vi "GetSignal.vi"(8 "error in (no error)":errorcluster, 11 "PmuTestFunctions in":refnum<class "PmuTestFunctions.lvclass">) -> (0 "error out":errorcluster, 2 "Signal":variant, 3 "PmuTestFunctions out":refnum<class "PmuTestFunctions.lvclass">)   [LabVIEW 2018, in "Functions.lvlib" / "PmuTestFunctions.lvclass"]
doc: "Gets the waveform, applies the gain and outputs a 2D array of the signal"
uses:
  PmuTestFunctions.lvclass
  X:/Projects/PMUCal/Modules/FGen/MemberClasses/FunctionBaseClass/FunctionBase.lvclass
  X:/Projects/PMUCal/Modules/FGen/MemberClasses/ArbitraryFunction/ArbitraryFunction.lvclass
  FunctionBaseClass/FunctionBase.lvclass/FunctionBase.ctl
  ArbitraryFunction/ArbitraryFunction.lvclass/ArbitraryFunction.ctl
  FunctionBaseClass/Accessors/Read Waveforms.vi
  ArbitraryFunction/Accessors/Read Arbs.vi
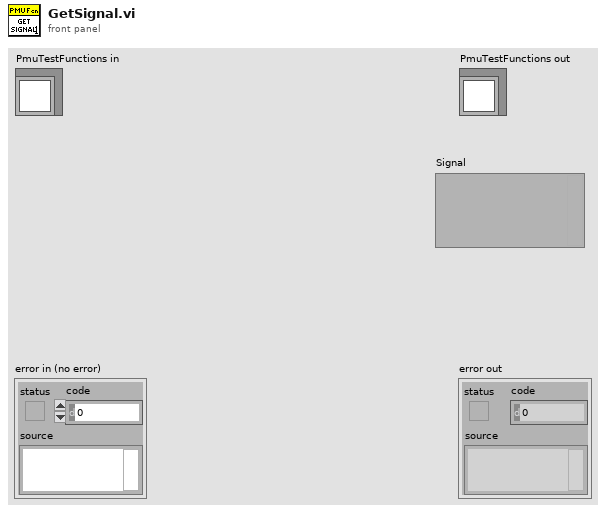
[diagram p1: front panel]
types:
  T1 = typedef "Functions.lvlib/ArbitraryFunction.lvclass/Arbitrary.ctl" = cluster{"Handle":string, "Size":i32, "Gain":dbl, "Offset":dbl, "Waveform":waveform(dbl)}
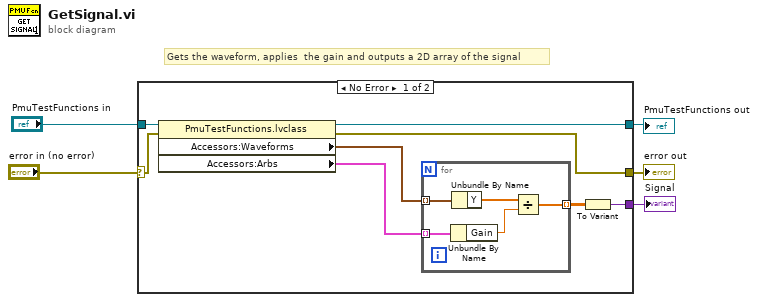
[diagram p0: block diagram]
diagram:
  # "Gets the waveform, applies  the gain and outputs a 2D array of the signal"
  n1 = case shown="No Error" "error in (no error)" {
    selector: "error in (no error)" -> [w12 w20]
    tunnel: "PmuTestFunctions in" -> [w13 w19]
    tunnel: [w8 w19] -> w3
    tunnel: [w7 _] -> w2
    tunnel: [w6 w20] -> w1
    frame No Error {
      n2 = property class="PmuTestFunctions.lvclass"(reference=w13, error in=w12) -> (reference out=w8:refnum<class "PmuTestFunctions.lvclass">, error out=w6:errorcluster, "Accessors:Waveforms"=w11:waveform(dbl)[], "Accessors:Arbs"=w10:T1[])
      n3 = for {
        tunnel: w11 -> [w18] mode=indexing
        tunnel: w10 -> [w17] mode=indexing
        tunnel: [w14] -> w9 mode=indexing
        n4 = Unbundle By Name(w17) -> ("Gain"=w15:dbl)
        n5 = Unbundle By Name(w18) -> ("Y"=w16:dbl[])
        n6 = Divide(x=w16, y=w15) -> (x/y=w14:dbl[])
      }
      n7 = To Variant(anything=w9) -> (Variant=w7:variant)
    }
    frame Error {
    }
  }
  "error out" <- w1
  "PmuTestFunctions out" <- w3
  "Signal" <- w2
